vi "Day03-04_지진 계측기.vi"() -> ()   [LabVIEW 2021]
panel:
  out "지진 검측 화면":dbl(graph)
  in  "감지 종료":bool
  in  "알람 리셋":bool
  in  "감지 시작":bool
  out "알람 발생":bool
  out "진도/발생 시간 기록":string
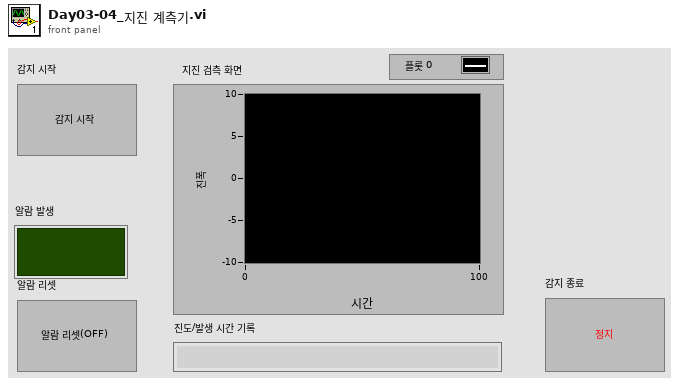
[diagram p1: front panel]
types:
  T1 = typedef "지진 계측기 상태 열거형 상수.ctl" = enum16{"초기화", "대기", "감지 시작", "알람 발생", "알람 리셋", "지진 검측 화면", "진도/발생 시간 기록", "LED", "정지"}
  T2 = cluster{"상태":T1, "감지 시작":bool, "알람 발생":bool, "알람 리셋":bool, "지진 검측 화면":bool, "진도/발생 시간 기록":string, "감지 종료":bool}
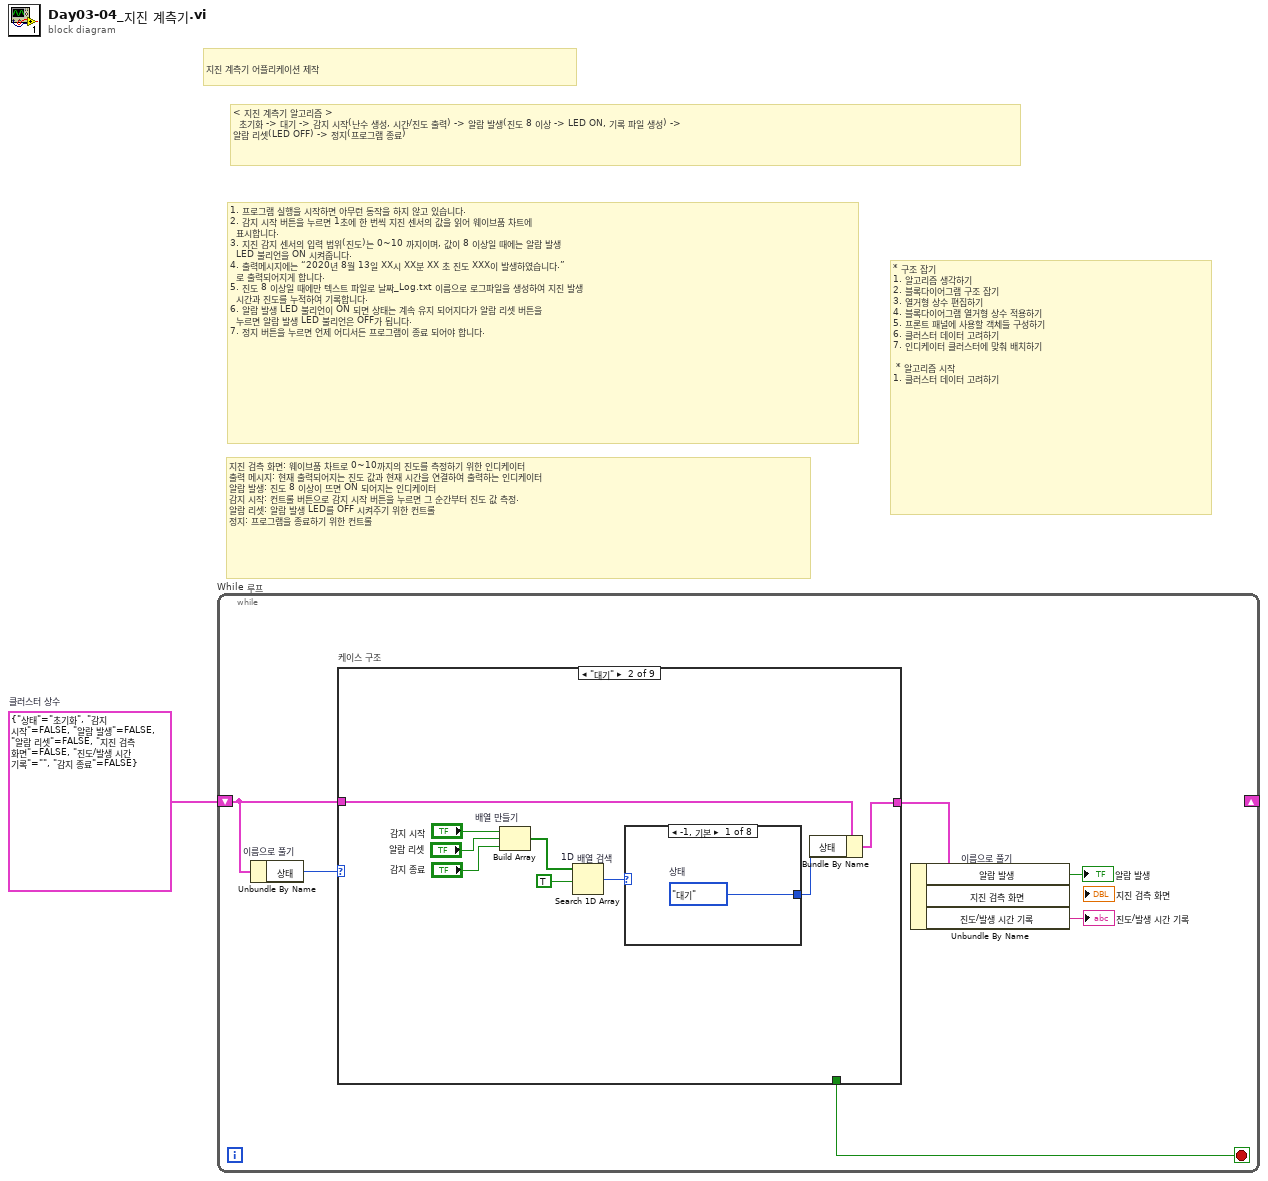
[diagram p0: block diagram]
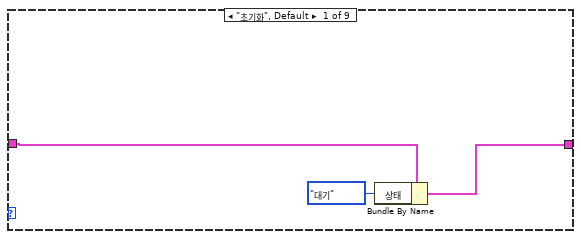
[diagram p2: hidden frame]
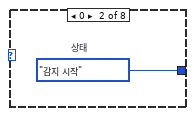
[diagram p3: hidden frame]
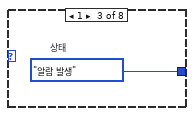
[diagram p4: hidden frame]
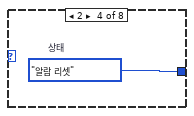
[diagram p5: hidden frame]
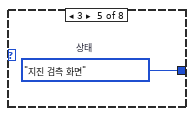
[diagram p6: hidden frame]
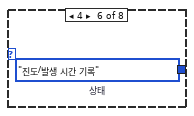
[diagram p7: hidden frame]
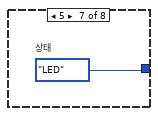
[diagram p8: hidden frame]
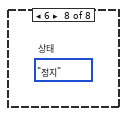
[diagram p9: hidden frame]
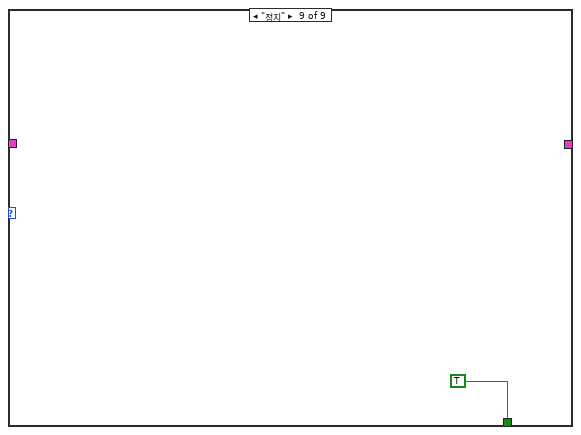
[diagram p16: hidden frame]
diagram:
  w1 = T2 {"상태"=enum."초기화", "감지 시작"=FALSE, "알람 발생"=FALSE, "알람 리셋"=FALSE, "지진 검측 화면"=FALSE, "진도/발생 시간 기록"="", "감지 종료"=FALSE}  # 클러스터 상수
  # "* 구조 잡기\n1. 알고리즘 생각하기\n2. 블록다이어그램 구조 잡기\n3. 열거형 상수 편집하기\n4. 블록다이어그램 열거형 상수 적용하기\n5. 프론트 패널에 사용할 객체들 구성하기\n6. 클러스터 데이터 고려하기\n7. 인디케이터 클러스터에 맞춰 배치하기\n\n * 알고리즘 시작\n1. 클러스터 데이터 고려하기"
  # "< 지진 계측기 알고리즘 >\n  초기화 -> 대기 -> 감지 시작(난수 생성, 시간/진도 출력) -> 알람 발생(진도 8 이상 -> LED ON, 기록 파일 생성) -> \n알람 리셋(LED OFF) -> 정지(프로그램 종료)"
  # "지진 계측기 어플리케이션 제작"
  # "지진 검측 화면: 웨이브품 차트로 0~10까지의 진도를 측정하기 위한 인디케이터\n출력 메시지: 현재 출력되어지는 진도 값과 현재 시간을 연결하여 출력하는 인디케이터\n알람 발생: 진도 8 이상이 뜨면 ON 되어지는 인디케이터\n감지 시작: 컨트롤 버튼으로 감지 시작 버튼을 누르면 그 순간부터 진도 값 측정.\n알람 리셋: 알람 발생 LED를 OFF 시켜주기 위한 컨트롤\n정지: 프로그램을 종료하기 위한 컨트롤"
  # "1. 프로그램 실행을 시작하면 아무런 동작을 하지 않고 있습니다.\n2. 감지 시작 버튼을 누르면 1초에 한 번씩 지진 센서의 값을 읽어 웨이브품 차트에 \n  표시합니다.\n3. 지진 감지 센서의 입력 범위(진도)는 0~10 까지이며, 값이 8 이상일 때에는 알람 발생\n  LED 불리언을 ON 시켜줍니다.\n4. 출력메시지에는 “2020년 8월 13일 XX시 XX분 XX 초 진도 XXX이 발생하였습니다.”\n  로 출력되어지게 합니다.\n5. 진도 8 이상일 때에만 텍스트 파일로 날짜_Log.txt 이름으로 로그파일을 생성하여 지진 발생\n  시간과 진도를 누적하여 기록합니다.\n6. 알람 발생 LED 불리언이 ON 되면 상태는 계속 유지 되어지다가 알람 리셋 버튼을\n  누르면 알람 발생 LED 불리언은 OFF가 됩니다.\n7. 정지 버튼을 누르면 언제 어디서든 프로그램이 종료 되어야 합니다."
  n1 = while "While 루프" {
    shift-right: _ -> [_]
    shift-left: w1 -> [w7]
    stop <- w3 stop-if-true
    n2 = Unbundle By Name "이름으로 풀기"(w7) -> ("상태"=w4:T1)
    n3 = case "케이스 구조" shown="\"대기\"" w4 {
      tunnel: w7 -> [w9 w19 _ _ _ _ _ _ _]
      tunnel: [w8 w18 _ _ _ _ _ _ _] -> w6
      tunnel: [_ _ _ _ _ _ _ _ TRUE] -> w3
      frame "초기화", Default {
        n4 = Bundle By Name(cluster=w9, "상태"=지진_계측기_상태_열거형_상수."대기") -> (w8:T2)
      }
      frame "대기" {
        n5 = Build Array "배열 만들기"("감지 시작", "알람 리셋", "감지 종료") -> (w12:bool[])
        n6 = Search 1D Array "1D 배열 검색"(1D array=w12, element=TRUE) -> (index of element=w14:i32)  [unwired: 1 in]
        n7 = case shown="-1, 기본" w14 {
          tunnel: [w20 w21 w22 w23 w24 _ w25 _] -> w11
          frame -1, Default {
            w20 = 지진_계측기_상태_열거형_상수."대기"  # 상태
          }
          frame 0 {
            w21 = 지진_계측기_상태_열거형_상수."감지 시작"  # 상태
          }
          frame 1 {
            w22 = 지진_계측기_상태_열거형_상수."알람 발생"  # 상태
          }
          frame 2 {
            w23 = 지진_계측기_상태_열거형_상수."알람 리셋"  # 상태
          }
          frame 3 {
            w24 = 지진_계측기_상태_열거형_상수."지진 검측 화면"  # 상태
          }
          frame 4 {
            (unwired) 지진_계측기_상태_열거형_상수."진도/발생 시간 기록"  # 상태
          }
          frame 5 {
            w25 = 지진_계측기_상태_열거형_상수."LED"  # 상태
          }
          frame 6 {
            (unwired) 지진_계측기_상태_열거형_상수."정지"  # 상태
          }
        }
        n8 = Bundle By Name(cluster=w19, "상태"=w11) -> (w18:T2)
      }
      frame "감지 시작" {
      }
      frame "알람 발생" {
      }
      frame "알람 리셋" {
      }
      frame "지진 검측 화면" {
      }
      frame "진도/발생 시간 기록" {
      }
      frame "LED" {
      }
      frame "정지" {
      }
    }
    n9 = Unbundle By Name "이름으로 풀기"(w6) -> ("알람 발생"=→"알람 발생":bool, "진도/발생 시간 기록"=→"진도/발생 시간 기록":string)  [unwired: 1 out]
  }
